vi "Read Analog Level.vi"(8 "error in (no error)":errorcluster, 9 "Channel (0: chA)":i32(ring) items=["chA", "chB"], 10 "Analyzer (0: A0)":i32(ring) items=["A0", "A1"], 11 "VISA resource name":refnum<visa-resource-name>) -> (0 "error out":errorcluster, 2 "Analog Level":dbl, 3 "VISA resource name out":refnum<visa-resource-name>)   [LabVIEW 2014, in "Stanford Research SR1.lvlib"]
doc: "Reads the Analog Generator Anaylzer level reading."
uses:
  Stanford Research SR1.lvlib
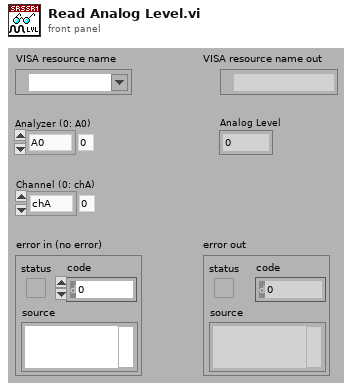
[diagram p1: front panel]
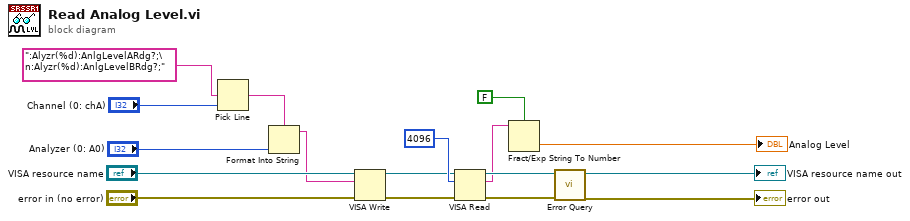
[diagram p0: block diagram]
diagram:
  n1 = Pick Line(multi-line string=":Alyzr(%d):AnlgLevelARdg?;\n:Alyzr(%d):AnlgLevelBRdg?;", line index="Channel (0: chA)") -> (output string=w3:string)  [unwired: 1 in]
  n2 = Format Into String(format string=w3, "Analyzer (0: A0)") -> (resulting string=w8:string)  [unwired: 2 in, 1 out]
  n3 = VISA Write(VISA resource name="VISA resource name", write buffer=w8, error in (no error)="error in (no error)") -> (VISA resource name out=w14:refnum<visa-resource-name>, error out=w13:errorcluster)  [unwired: 1 out]
  n4 = VISA Read(VISA resource name=w14, byte count=u32 4096, error in (no error)=w13) -> (VISA resource name out=w12:refnum<visa-resource-name>, read buffer=w7:string, error out=w11:errorcluster)  [unwired: 1 out]
  n5 = Fract/Exp String To Number(use system decimal point (T)=FALSE, string=w7) -> (number=→"Analog Level":dbl)  [unwired: 2 in, 1 out]
  n6 = call "Error Query.vi"("error in (no error)"=w11, "VISA resource name"=w12) -> ("error out"=→"error out":errorcluster, "VISA resource name out"=→"VISA resource name out":refnum<visa-resource-name>)  [unwired: 6 in, 2 out]
